vi "Append Waveforms Sweep.vi"(8 "error in (no error)":errorcluster, 9 "AI":waveform(dbl)[](array[waveform]), 10 "AO":waveform(dbl)[](array[waveform]), 11 "IVSweepResults []":T1(array[cluster])) -> (0 "error out":errorcluster, 3 "Array":T1(array[cluster]))   [LabVIEW 2016, in "Lockin.DAQ.lvclass"]
uses:
  Lockin.DAQ.lvclass
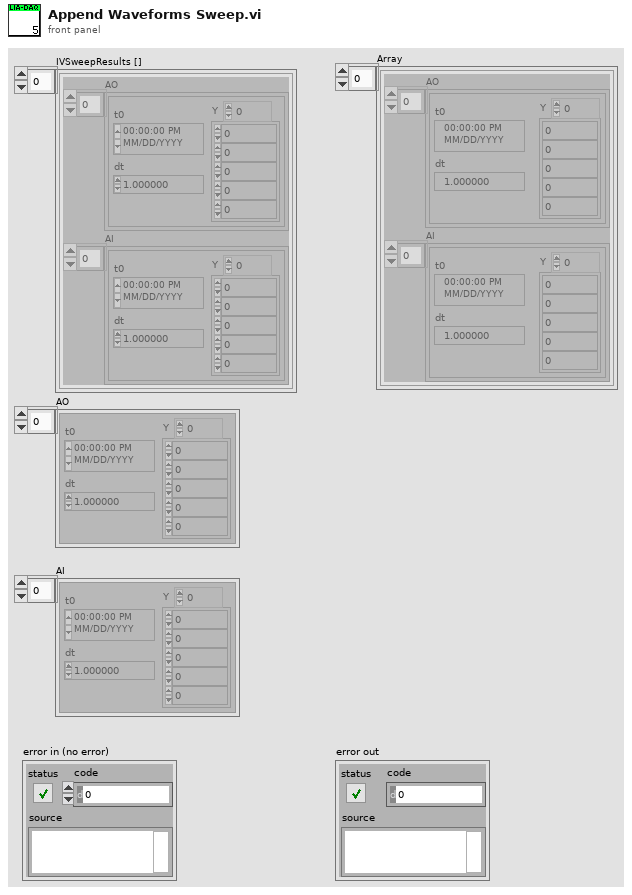
[diagram p1: front panel]
types:
  T1 = cluster{"AO":waveform(dbl)[], "AI":waveform(dbl)[]}[]
  T2 = cluster{"AO":waveform(dbl)[], "AI":waveform(dbl)[]}
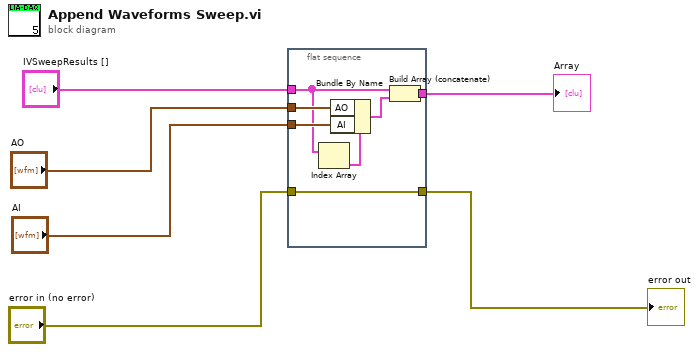
[diagram p0: block diagram]
diagram:
  n1 = flat-sequence {
    tunnel: "AO" -> [w13]
    tunnel: "AI" -> [w12]
    tunnel: [w10] -> w4
    tunnel: "IVSweepResults []" -> [w8]
    tunnel: "error in (no error)" -> [w7]
    tunnel: [w7] -> w6
    frame #0 {
      n2 = Index Array(array=w8) -> (element=w11:T2)  [unwired: 1 in]
      n3 = Bundle By Name(cluster=w11, "AO"=w13, "AI"=w12) -> (w9:T2)
      n4 = Build Array (concatenate)(w8, w9) -> (w10:T1)
    }
  }
  "error out" <- w6
  "Array" <- w4
